vi "VR_Data_Collection.vi"() -> ()   [LabVIEW 2022 SP3]
panel:
  out "Numeric":dbl
  out "Waveform Graph":dynamicdata(graph)
  out "XY Graph":cluster{"Y":dbl[], "Y":dbl[]}[](graph)
  in  "stop":bool
  out "VR":dbl(knob) scale=-0.02..0.02
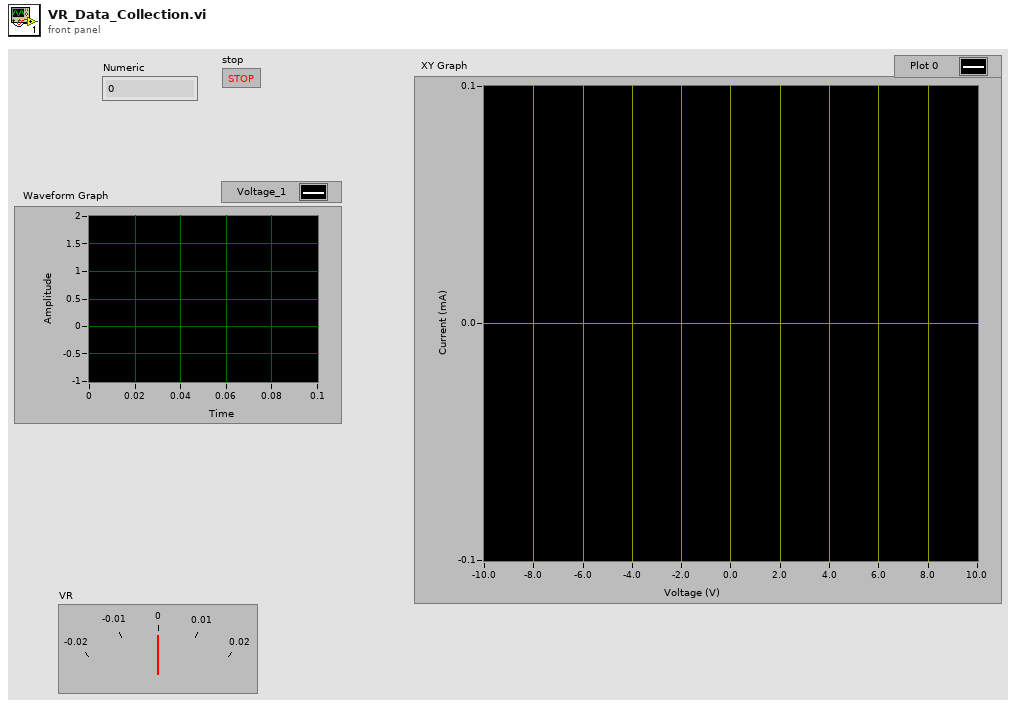
[diagram p1: front panel]
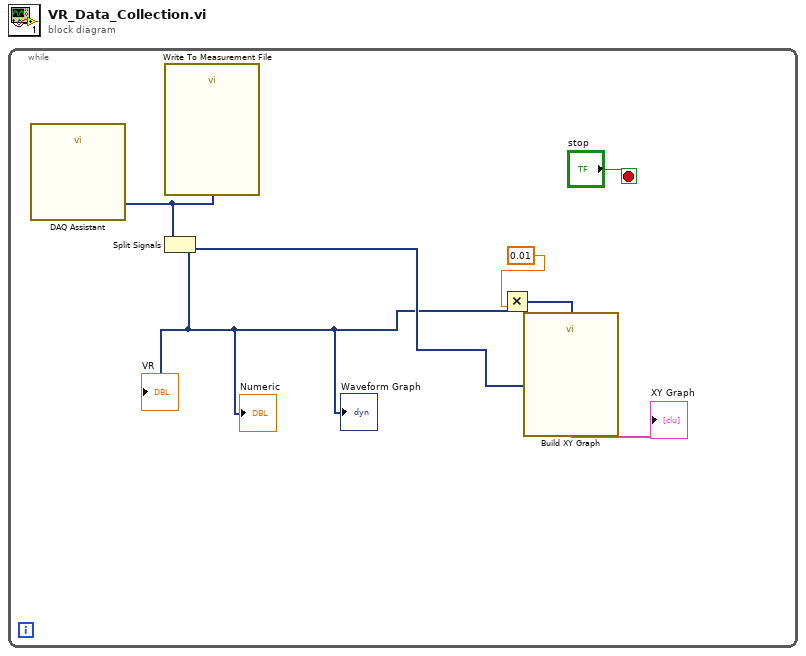
[diagram p0: block diagram]
diagram:
  n1 = while {
    stop <- "stop" stop-if-true
    n2 = call "DAQ Assistant"() -> ("data"=w2:dynamicdata)  [unwired: 17 in, 2 out]
    n3 = call "Write To Measurement File"("Signals"=w2) -> ()  [unwired: 16 in, 3 out]
    n4 = Split Signals(w2) -> (w1:dynamicdata, w3:dynamicdata)  [unwired: 2 in]
    "VR" <- w1
    "Waveform Graph" <- w1
    "Numeric" <- w1
    n5 = Multiply(x=w1, y=0.01) -> (x*y=w4:dynamicdata)
    n6 = call "Build XY Graph"("Y Input"=w4, "X Input"=w3) -> ("XY Graph"=→"XY Graph":cluster{"X":dbl[], "Y":dbl[]}[])  [unwired: 8 in, 1 out]
  }
